vi "obj_ClientSrv Connection State.vi"(0 "method (get state)":T2=enum."get state", 5 "machine{connect}/VI{get state} name (local/no path resolution)":string, 7 "port number in (3363)":u32=3363, 9 "observer digest":string, 11 "error in (no error)":errorcluster) -> (2 "server access":T1, 3 "local?":bool, 4 "server app ref":refnum<vi>, 6 "resolved server path":path, 8 "observer certificate":string, 10 "connected?":bool, 14 "server":string, 15 "error out":errorcluster)   [LabVIEW 2012]
doc: "This client-side object holds state pertaining to the client's connection with the remote server application. The client can connect only to a single server at any one time."
uses:
  typedefs/t_ClientSrv Connection State Methods.ctl
  served/ClientSrv Server Access_srv.ctl
  typedefs/t_ClientSrv Server Access Methods.ctl
  typedefs/t_ClientSrv Access Levels.ctl
  subvis/private/glb_ClientSrv Globals.vi
  library/glb_Library Configuration Globals.vi
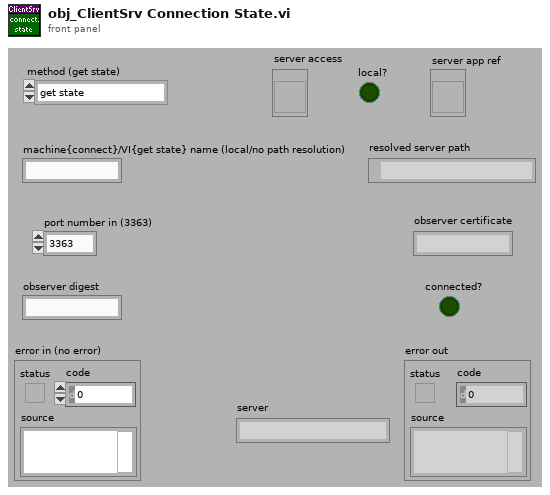
[diagram p1: front panel]
types:
  T1 = typedef "ClientSrv Server Access_srv.ctl" = refnum<vi>
  T2 = typedef "t_ClientSrv Connection State Methods.ctl" = enum16{"connect", "get state", "disconnect"}
  T3 = typedef "t_ClientSrv Access Levels.ctl" = enum16{"observer", "operator", "local"}
  T4 = typedef "t_ClientSrv Server Access Methods.ctl" = enum16{"validate access", "test access", "release access", "get name"}
  T5 = enum32{"invalid app kind", "Development System", "Run Time System", "Student Edition", "Embedded LabVIEW", "Evaluation", "Custom"}
  T6 = typedef "et_Library Error Code Enum.ctl" = enum32{"No error", "Argument error", "Memory is full", "Out of zone", "End of file", "File already open", "Generic file I/O error", "File not found", "File permission error", "Disk is full", "Duplicate path", "Too many files open", "System feature not enabled", "Resource file not found", "Cannot add resource", "Resource not found", "Image not found", "Image memory error", "Pen does not exist", "Config type invalid", "Config token not found", "Config parse error", "Config memory error", "Bad external code format", "Bad external code offset", "External code not present", "Null window", "Destroy window error", "Null menu", "Print aborted", "Bad print record", "Print driver error", "Windows error during printing", "Memory error during printing", "Print dialog error", "Generic print error", "Invalid device refnum", "Device not found", "Device parameter error", "Device unit error", "Cannot open device", "Device call aborted", "Generic error", "Cancelled by user", "Object ID too low", "Object ID too high", "Object not in heap", "Unknown heap", "Unknown object (invalid DefProc)", "Unknown object (DefProc not in table)", "Message out of range", "Invalid (null) method", "Unknown message", "Manager call not supported", "Bad address", "Network operation in progress", "Network operation timed out", "Connection is busy", "Network attribute not supported", "Network error", "Address in use", "System out of memory", "Connection aborted", "Connection refused", "Not connected", "Already connected", "Connection closed", "Initialization error (interapplication manager)", "Bad occurrence", "Wait on unbound occurrence handler", "Occurrence queue overflow", "Datalog type conflict", "Unused", "Unrecognized type (interapplication manager)", "Memory corrupt", "Failed to make temporary DLL", "Old CIN version", "Drag socket not found", "Failed to load drop-object", "Failed to register OLE object", "Failed to release OLE object", "Format specifier type mismatch", "Unknown format specifier", "Too few format specifiers", "Too many format specifiers", "Scan failed", "Newer CIN version", "Error converting to variant", "Runtime menu error", "Password tampered", "Variant attribute not found", "Incompatible variant data type", "Event data is not available", "Event Store is not present", "Occurrence is not found", "Event Queue is not created", "Event info is not available in the type library", "Refnum passed is NULL", "Error retrieving Class GUID", "Error retrieving CoClass GUID", "Error retrieving TypeLib GUID.", "Bad built application magic bytes.", "Specific driver is different from the specific driver associated with the Logical Name.", "There is no session opened to the class driver.", "Max Error", "MAX - Error with config objects", "MAX - Error loading configuration", "MAX - Group not supported", "Singlecast connections can not send to multicast addresses.", "Multicast connections can not send to singlecast addresses.", "Specified IP address not in multicast address range.", "Attempt to write to read-only multicast connection.", "Attempt to read from write-only multicast connection.", "The buffer used to receive a datagram was smaller than the datagram itself", "Error code not enumerated"}
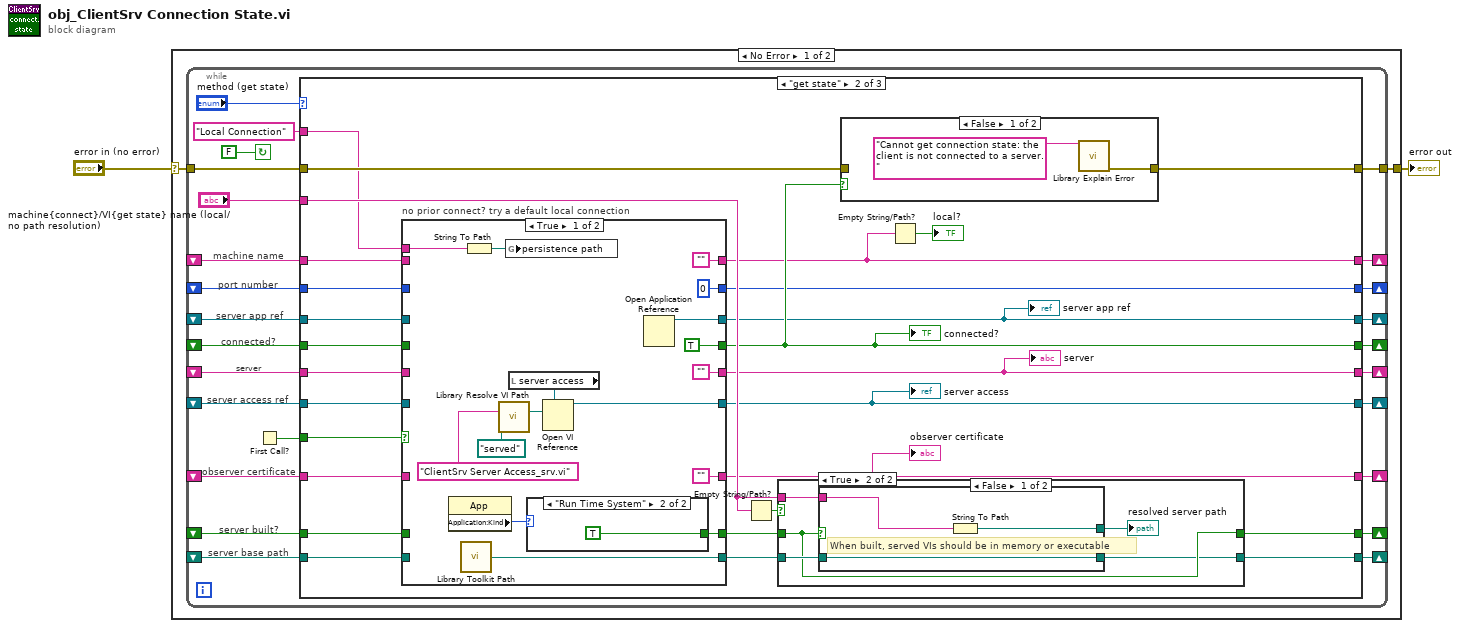
[diagram p0: block diagram]
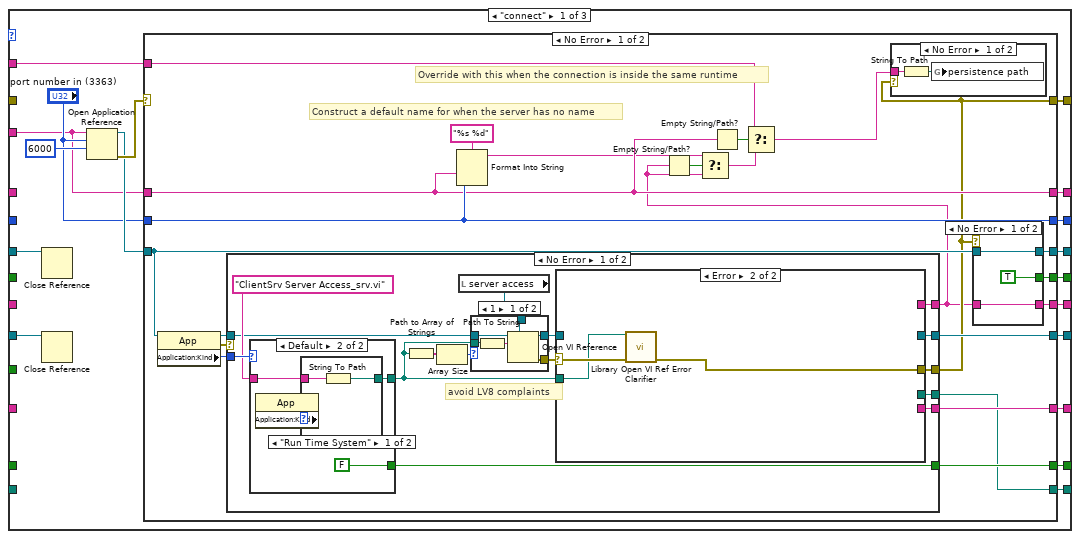
[diagram p2: hidden frame]
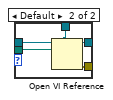
[diagram p4: hidden frame]
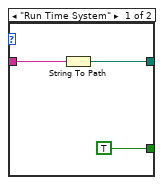
[diagram p5: hidden frame]
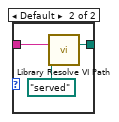
[diagram p6: hidden frame]
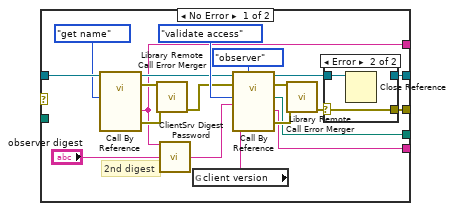
[diagram p7: hidden frame]
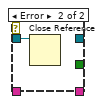
[diagram p10: hidden frame]
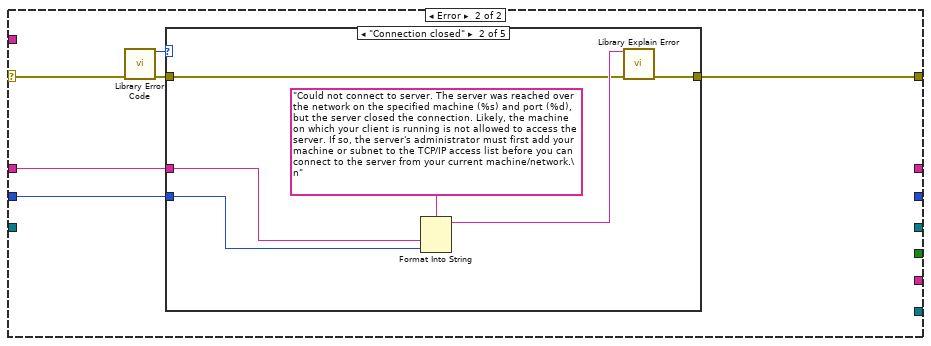
[diagram p11: hidden frame]
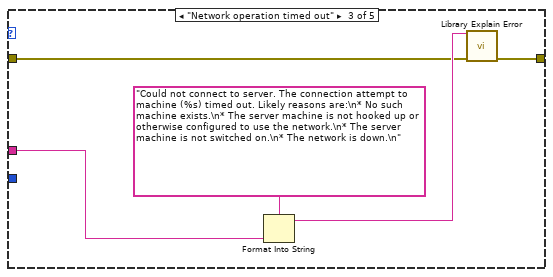
[diagram p13: hidden frame]
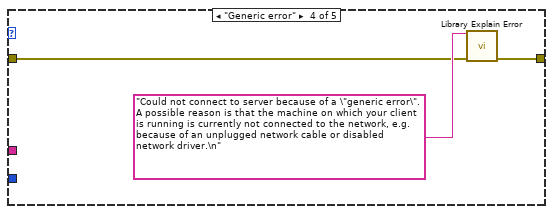
[diagram p14: hidden frame]
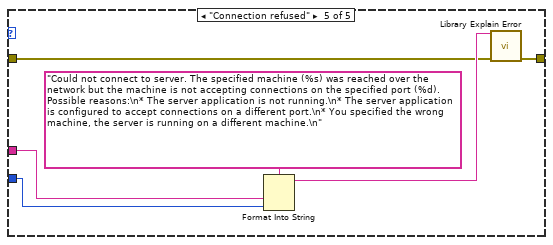
[diagram p15: hidden frame]
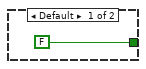
[diagram p16: hidden frame]
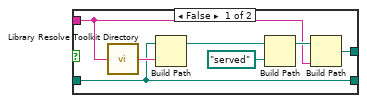
[diagram p18: hidden frame]
diagram:
  n1 = case shown="No Error" "error in (no error)" {
    selector: "error in (no error)" -> [w4 w257]
    tunnel: [w3 w257] -> w1
    frame No Error {
      n2 = while {
        shift-right: [w29] -> _
        shift-left: _ -> [w28]
        shift-right: [w26] -> _
        shift-left: _ -> [w27]
        tunnel: w4 -> [w25]
        tunnel: [w24] -> w3
        shift-right: [w22] -> _
        shift-left: _ -> [w23]
        shift-right: [w20] -> _
        shift-left: _ -> [w21]
        shift-right: [w18] -> _
        shift-left: _ -> [w19]
        shift-right: [w14] -> _
        shift-left: _ -> [w15]
        shift-right: [w12] -> _
        shift-left: _ -> [w13]
        shift-right: [w11] -> _
        shift-left: _ -> [w10]
        shift-right: [w8] -> _
        shift-left: _ -> [w9]
        stop <- FALSE continue-if-true
        # "server base path"
        # "server built?"
        # "observer certificate"
        # "server access ref"
        # "server"
        # "port number"
        # "connected?"
        # "server app ref"
        # "machine name"
        n3 = First Call?() -> (First Call?: T/F=w6:bool)
        n4 = case shown="\"get state\"" "method (get state)" {
          tunnel: w28 -> [_ w192 _]
          tunnel: [w45 w171 ""] -> w29
          tunnel: [w44 w173 refnum<k0> refnum] -> w26
          tunnel: w27 -> [w42 w190 w256]
          tunnel: w25 -> [_ w194 w251]
          tunnel: [w40 w195 w251] -> w24
          tunnel: w23 -> [_ w189 _]
          tunnel: [w43 w174 FALSE] -> w22
          tunnel: w21 -> [_ w191 _]
          tunnel: [w39 w172 u32 0 ("port number in (3363)")] -> w20
          tunnel: w19 -> [_ w188 _]
          tunnel: [w37 w175 ""] -> w18
          tunnel: w15 -> [w36 w187 w249]
          tunnel: [w35 w176 refnum<k0> refnum] -> w14
          tunnel: w13 -> [_ w186 _]
          tunnel: [w34 w177 ""] -> w12
          tunnel: [w33 w181 FALSE] -> w11
          tunnel: w10 -> [_ w185 _]
          tunnel: w9 -> [_ w184 _]
          tunnel: [w32 w180 path ""] -> w8
          tunnel: "machine{connect}/VI{get state} name (local/no path resolution)" -> [w31 w182 _]
          tunnel: w6 -> [_ w170 _]
          tunnel: "Local Connection" -> [w30 w169 w243]
          frame "connect" {
            n5 = Close Reference(reference=w42) -> ()  [unwired: 1 in, 1 out]
            n6 = Close Reference(reference=w36) -> ()  [unwired: 1 in, 1 out]
            n7 = Open Application Reference(9:6000 ("timeout ms (60000)"), 10:"port number in (3363)", 11:w31) -> (0:w47:errorcluster, 3:w46:refnum<vi>)  [unwired: 1 in]
            n8 = case shown="No Error" w47 {
              selector: w47 -> [_ w144]
              tunnel: w31 -> [w67 w146]
              tunnel: w46 -> [w59 _]
              tunnel: [w67 _] -> w45
              tunnel: [w64 _] -> w44
              tunnel: [w63 _] -> w43
              tunnel: [w52 w147] -> w40
              tunnel: "port number in (3363)" -> [w68 w145]
              tunnel: [w68 _] -> w39
              tunnel: [w50 _] -> w37
              tunnel: [w65 _] -> w35
              tunnel: [w55 _] -> w34
              tunnel: [w54 _] -> w33
              tunnel: [w53 _] -> w32
              tunnel: w30 -> [w51 _]
              frame No Error {
                # "Override with this when the connection is inside the same runtime"
                # "Construct a default name for when the server has no name"
                n9 = property class="App"(reference=w59) -> (reference out=w58:refnum<vi>, error out=w57:errorcluster, "Application:Kind"=w56:T5)  [unwired: 1 in]
                n10 = case shown="No Error" w57 {
                  selector: w57 -> [_ w137]
                  tunnel: [w86 _] -> w65
                  tunnel: [w85 w137] -> w52
                  tunnel: [w84 _] -> w55
                  tunnel: [w83 _] -> w48
                  tunnel: w58 -> [w73 _]
                  tunnel: w56 -> [w82 _]
                  tunnel: [w80 _] -> w54
                  tunnel: [w79 _] -> w53
                  frame No Error {
                    # "avoid LV8 complaints"
                    n11 = case shown="Default" w82 {
                      tunnel: [w98 w102] -> w72
                      tunnel: [TRUE FALSE] -> w80
                      tunnel: "ClientSrv Server Access_srv.vi" -> [w99 w104]
                      frame "Run Time System" {
                        n12 = String To Path(string=w99) -> (path=w98:path)
                      }
                      frame Default {
                        n13 = property class="App"() -> ("Application:Kind"=w101:T5)  [unwired: 2 in, 2 out]
                        n14 = case shown="\"Run Time System\"" w101 {
                          tunnel: w104 -> [w106 w108]
                          tunnel: [w105 w107] -> w102
                          frame "Run Time System" {
                            n15 = String To Path(string=w106) -> (path=w105:path)
                          }
                          frame Default {
                            n16 = call "Library Resolve VI Path.vi"("VI name"=w108, "sub path of toolkit (none)"=path "served" ("subdirectory of tree (none)")) -> ("VI path"=w107:path)  [unwired: 13 in]
                          }
                        }
                      }
                    }
                    n17 = Path to Array of Strings(0:w72) -> (2:w78:string[])  [unwired: 1 out]
                    n18 = Array Size(array=w78) -> (size(s)=w77:i32)
                    n19 = local read "server access"() -> (w74:T1)
                    n20 = case shown="1" w77 {
                      tunnel: w72 -> [w92 w97]
                      tunnel: w73 -> [w90 w96]
                      tunnel: [w89 w95] -> w75
                      tunnel: [w87 w94] -> w76
                      tunnel: w74 -> [w88 w93]
                      frame 1 {
                        n21 = Path To String(path=w92) -> (string=w91:string)
                        n22 = Open VI Reference(type specifier VI Refnum (for type only)=w88, application reference (local)=w90, vi path=w91) -> (vi reference=w89:T1, error out=w87:errorcluster)  [unwired: 3 in]
                      }
                      frame Default {
                        n23 = Open VI Reference(type specifier VI Refnum (for type only)=w93, application reference (local)=w96, vi path=w97) -> (vi reference=w95:T1, error out=w94:errorcluster)  [unwired: 3 in]
                      }
                    }
                    n24 = case shown="Error" w76 {
                      selector: w76 -> [_ w136]
                      tunnel: w75 -> [w129 _]
                      tunnel: [w122 _] -> w86
                      tunnel: [w121 w134] -> w85
                      tunnel: [w112 _] -> w83
                      tunnel: [w118 _] -> w84
                      tunnel: w72 -> [_ w135]
                      tunnel: [w114 _] -> w79
                      frame No Error {
                        # "2nd digest"
                        n25 = call-by-ref "?"(reference=w129, "method"=t_ClientSrv_Server_Access_Methods."get name") -> (reference out=w120:T1, error out=w127:errorcluster, "certificate/name out"=w112:string, 15:"error out"=w126:errorcluster)  [unwired: 13 in, 1 out]
                        n26 = call "Library Remote Call Error Merger.vi"("call by reference node error"=w127, "called VI error (no error)"=w126) -> ("error out"=w117:errorcluster)  [unwired: 13 in]
                        n27 = call "ClientSrv Digest Password.vi"("server name (none)"=w112, "password"="observer digest") -> ("SHA-1 digest"=w113:string)  [unwired: 13 in]
                        n28 = global read "glb_ClientSrv Globals.vi" "client version"() -> (w110:string)
                        n29 = call-by-ref "?"(reference=w120, error in=w117, "method"=t_ClientSrv_Server_Access_Methods."validate access", "access level"=t_ClientSrv_Access_Levels."observer", "digest"=w113, "client version"=w110) -> (reference out=w119:T1, error out=w125:errorcluster, "server toolkit path"=w114:path, "certificate/name out"=w118:string, 15:"error out"=w123:errorcluster)  [unwired: 9 in]
                        n30 = call "Library Remote Call Error Merger.vi"("call by reference node error"=w125, "called VI error (no error)"=w123) -> ("error out"=w116:errorcluster)  [unwired: 13 in]
                        n31 = case shown="Error" w116 {
                          selector: w116 -> [w130 w132]
                          tunnel: w119 -> [w131 w133]
                          tunnel: [w131 _] -> w122
                          tunnel: [w130 w132] -> w121
                          frame No Error {
                          }
                          frame Error {
                            n32 = Close Reference(reference=w133) -> ()  [unwired: 1 in, 1 out]
                          }
                        }
                      }
                      frame Error {
                        n33 = call "Library Open VI Ref Error Clarifier.vi"("VI path"=w135, "called VI error (no error)"=w136) -> ("error out"=w134:errorcluster)  [unwired: 13 in]
                      }
                    }
                  }
                  frame Error {
                  }
                }
                n34 = Format Into String(format string="%s %d", w67, w68) -> (resulting string=w61:string)  [unwired: 2 in, 1 out]
                n35 = Empty String/Path?(string/path=w48) -> (empty?=w62:bool)
                n36 = Select(t=w61, s=w62, f=w48) -> (s? t:f=w60:string)
                n37 = Empty String/Path?(string/path=w67) -> (empty?=w66:bool)
                n38 = Select(t=w51, s=w66, f=w60) -> (s? t:f=w49:string)
                n39 = case shown="No Error" w52 {
                  tunnel: w49 -> [w70 _]
                  frame No Error {
                    n40 = String To Path(string=w70) -> (path=w71:path)
                    n41 = global write "glb_Library Configuration Globals.vi" "persistence path"(w71) -> ()
                  }
                  frame Error {
                  }
                }
                n42 = case shown="No Error" w52 {
                  tunnel: w59 -> [w140 w141]
                  tunnel: [w140 _] -> w64
                  tunnel: [TRUE _] -> w63
                  tunnel: w48 -> [w138 _]
                  tunnel: [w138 _] -> w50
                  frame No Error {
                  }
                  frame Error {
                    n43 = Close Reference(reference=w141) -> ()  [unwired: 1 in, 1 out]
                  }
                }
              }
              frame Error {
                n44 = call "Library Error Code.vi"("error"=w144) -> ("error code enum"=w142:T6, "dup error"=w143:errorcluster)  [unwired: 12 in, 1 out]
                n45 = case shown="\"Connection closed\"" w142 {
                  tunnel: w143 -> [w148 w149 w155 w160 w163]
                  tunnel: [w148 w154 w159 w162 w168] -> w147
                  tunnel: w146 -> [_ w153 w158 _ w167]
                  tunnel: w145 -> [_ w152 _ _ w166]
                  frame Default {
                  }
                  frame "Connection closed" {
                    n46 = Format Into String(format string="Could not connect to server. The server was reached over the network on the specified machine (%s) and port (%d), but the server closed the connection. Likely, the machine on which your client is running is not allowed to access the server. If so, the server's administrator must first add your machine or subnet to the TCP/IP access list before you can connect to the server from your current machine/network.\n" ("explanation"), w153, w152) -> (resulting string=w151:string)  [unwired: 2 in, 1 out]
                    n47 = call "Library Explain Error.vi"("explanation prefix (none)"=w151, "error in (no error)"=w149) -> ("explained error"=w154:errorcluster)  [unwired: 13 in]
                  }
                  frame "Network operation timed out" {
                    n48 = Format Into String(format string="Could not connect to server. The connection attempt to machine (%s) timed out. Likely reasons are:\n* No such machine exists.\n* The server machine is not hooked up or otherwise configured to use the network.\n* The server machine is not switched on.\n* The network is down.\n" ("explanation"), w158) -> (resulting string=w157:string)  [unwired: 2 in, 1 out]
                    n49 = call "Library Explain Error.vi"("explanation prefix (none)"=w157, "error in (no error)"=w155) -> ("explained error"=w159:errorcluster)  [unwired: 13 in]
                  }
                  frame "Generic error" {
                    n50 = call "Library Explain Error.vi"("explanation prefix (none)"="Could not connect to server because of a \"generic error\". A possible reason is that the machine on which your client is running is currently not connected to the network, e.g. because of an unplugged network cable or disabled network driver.\n" ("explanation"), "error in (no error)"=w160) -> ("explained error"=w162:errorcluster)  [unwired: 13 in]
                  }
                  frame "Connection refused" {
                    n51 = Format Into String(format string="Could not connect to server. The specified machine (%s) was reached over the network but the machine is not accepting connections on the specified port (%d). Possible reasons:\n* The server application is not running.\n* The server application is configured to accept connections on a different port.\n* You specified the wrong machine, the server is running on a different machine.\n" ("explanation"), w167, w166) -> (resulting string=w165:string)  [unwired: 2 in, 1 out]
                    n52 = call "Library Explain Error.vi"("explanation prefix (none)"=w165, "error in (no error)"=w163) -> ("explained error"=w168:errorcluster)  [unwired: 13 in]
                  }
                }
              }
            }
          }
          frame "get state" {
            n53 = case "no prior connect? try a default local connection" shown="True" w170 {
              tunnel: w192 -> [_ w222]
              tunnel: w191 -> [_ w221]
              tunnel: w190 -> [_ w220]
              tunnel: w189 -> [_ w219]
              tunnel: w188 -> [_ w218]
              tunnel: w187 -> [_ w217]
              tunnel: w186 -> [_ w216]
              tunnel: w185 -> [_ w215]
              tunnel: w184 -> [_ w214]
              tunnel: [w209 w214] -> w179
              tunnel: [w207 w215] -> w178
              tunnel: ["" ("certificate out") w216] -> w177
              tunnel: [w202 w217] -> w176
              tunnel: ["" ("machine{connect}/VI{get state} name (local/no path resolution)") w218] -> w175
              tunnel: [TRUE w219] -> w174
              tunnel: [w211 w220] -> w173
              tunnel: [u32 0 ("port number in (3363)") w221] -> w172
              tunnel: ["" ("machine{connect}/VI{get state} name (local/no path resolution)") w222] -> w171
              tunnel: w169 -> [w196 _]
              frame True {
                n54 = property class="App"() -> ("Application:Kind"=w208:T5)  [unwired: 2 in, 2 out]
                n55 = call "Library Toolkit Path.vi"() -> ("absolute toolkit path"=w209:path)  [unwired: 15 in]
                n56 = String To Path(string=w196) -> (path=w197:path)
                n57 = call "Library Resolve VI Path.vi"("VI name"="ClientSrv Server Access_srv.vi", "sub path of toolkit (none)"=path "served" ("subdirectory of tree (none)")) -> ("VI path"=w203:path)  [unwired: 13 in]
                n58 = global write "glb_Library Configuration Globals.vi" "persistence path"(w197) -> ()
                n59 = local read "server access"() -> (w205:T1)
                n60 = case shown="\"Run Time System\"" w208 {
                  tunnel: [FALSE TRUE] -> w207
                  frame Default {
                  }
                  frame "Run Time System" {
                  }
                }
                n61 = Open VI Reference(type specifier VI Refnum (for type only)=w205, vi path=w203) -> (vi reference=w202:T1)  [unwired: 4 in, 1 out]
                n62 = Open Application Reference() -> (3:w211:refnum<vi>)  [unwired: 4 in, 1 out]
              }
              frame False {
              }
            }
            "connected?" <- w174
            "server" <- w175
            "observer certificate" <- w177
            "server app ref" <- w173
            "server access" <- w176
            n63 = Empty String/Path?(string/path=w182) -> (empty?=w183:bool)
            n64 = case shown="False" w183 {
              tunnel: w178 -> [w224 w239]
              tunnel: w179 -> [w227 w238]
              tunnel: w182 -> [w225 _]
              tunnel: [w224 w239] -> w181
              tunnel: [w223 w238] -> w180
              frame False {
                n65 = case shown="True" w224 {
                  tunnel: w225 -> [w229 w237]
                  tunnel: [w230 w236] -> w226
                  tunnel: w227 -> [w228 w235]
                  tunnel: [w228 w235] -> w223
                  frame False {
                    n66 = call "Library Resolve Toolkit Directory.vi"("VI name"=w229) -> ("toolkit directory"=w234:string)
                    n67 = Build Path(base path=w228, name or relative path=w234) -> (appended path=w233:path)
                    n68 = Build Path(base path=w233, name or relative path=path "served") -> (appended path=w231:path)
                    n69 = Build Path(base path=w231, name or relative path=w229) -> (appended path=w230:path)
                  }
                  frame True {
                    # "When built, served VIs should be in memory or executable"
                    n70 = String To Path(string=w237) -> (path=w236:path)
                  }
                }
                "resolved server path" <- w226
              }
              frame True {
              }
            }
            n71 = case shown="False" w174 {
              tunnel: [w241 w242] -> w195
              tunnel: w194 -> [_ w242]
              frame False {
                n72 = call "Library Explain Error.vi"("explanation prefix (none)"="Cannot get connection state: the client is not connected to a server." ("explanation")) -> ("explained error"=w241:errorcluster)  [unwired: 14 in]
              }
              frame True {
              }
            }
            n73 = Empty String/Path?(string/path=w171) -> (empty?=→"local?":bool)
          }
          frame "disconnect" {
            # "Do not disconnect until all clients windows have closed or else the persistence data gets misplaced."
            n74 = String To Path(string=w243) -> (path=w244:path)
            n75 = global write "glb_Library Configuration Globals.vi" "persistence path"(w244) -> ()
            n76 = Close Reference(reference=w256) -> ()  [unwired: 1 in, 1 out]
            n77 = Close Reference(reference=w249) -> ()  [unwired: 1 in, 1 out]
          }
        }
      }
    }
    frame Error {
    }
  }
  "error out" <- w1
